vi "Programmer.vi"() -> ()   [LabVIEW 2017]
uses:
  <vilib>/Utility/config.llb/Read Key (String).vi
  <vilib>/Instr/_visa.llb/VISA Configure Serial Port (Instr).vi
  <vilib>/Utility/config.llb/NI_LVConfig.lvlib
panel:
  in  "CmdBaud":u32(ring)=230400 items=["4800"=4800, "9600"=9600, "19200"=19200, "38400"=38400, "57600"=57600, "115200"=115200, "230400"=230400, "460800"=460800, "921600"=921600]
  in  "FlashBaud":u32(ring)=230400 items=["4800"=4800, "9600"=9600, "19200"=19200, "38400"=38400, "57600"=57600, "115200"=115200, "230400"=230400, "460800"=460800, "921600"=921600]
  in  "COM Port":refnum<visa-resource-name>="COM4"
  out "RxMessage":u8[](array[numeric])
  out "LoaderCmdCount":i32
  in  "ClearPannel":bool
  in  "Read":bool
  out "Timeout?":bool
  out "Error List":string
  in  "Start":bool
  out "HeaderCount":i32
  out "AutoBaudCount":i32
  in  "File Path Control":path
  in  "Connect":bool
  in  "Stop Button":bool
  out "Rx":u64
  out "Tx":u64
  # "Ver 1.0.7"
  # "© Redler Technologies. All Rights Reserved"
  # "16:20:49 Operation stopped by user\n16:20:15 Driver Version: 20215\n16:20:14 Getting Driver version...\n16:20:14 Program success !\n16:20:13 Program start...\n16:20:13 Erase success !\n16:20:08 Erase start...\n16:20:08 Autobaud handshake success !\n16:20:05 Sending autobaud operation...\n16:20:05 Getting Driver version failed !\n16:20:02 Getting Driver version...\n16:20:02 Openning COM Port success !\n16:20:01 Openning COM Port..."
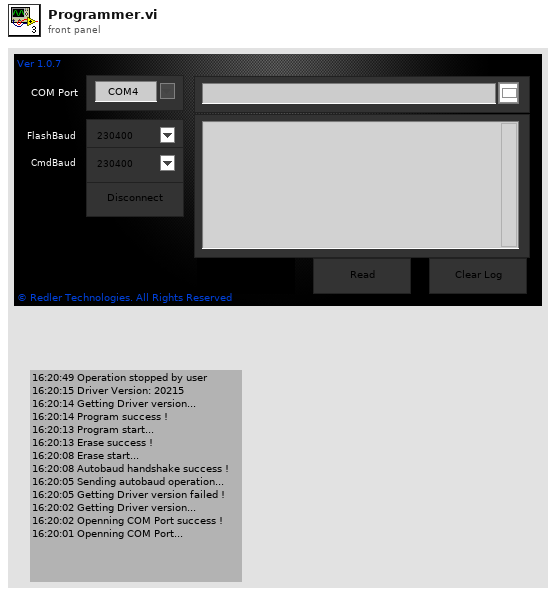
[diagram p1: front panel]
types:
  T1 = typedef "Semaphore RefNum" = refnum<k1>
  T2 = cluster{"Send Debug":string, "idx":i32, "DataType":enum8{"Int", " float"}, "Cmd id":u16, "Get/Set":enum8{"Set", "Get"}}
  T3 = cluster{"Send Debug":string, "idx":u16, "DataType":enum8{"Int", " float"}, "Cmd id":u16, "Get/Set":enum8{"Set", "Get"}}
  T4 = cluster{"Send Debug":string, "idx":u16, "DataType":enum8{"Int", " float"}, "Cmd id":u16, "Get/Set":enum8{"Set", "Get"}}[]
  T5 = typedef "NI_LVConfig.lvlib/Config Data RefNum.ctl" = refnum<k1>
  T6 = cluster{"Data":string, "idx":u16, "DataType":enum8{"Int", " float"}, "Cmd id":u16, "Get/Set":enum8{"Set", "Get"}}
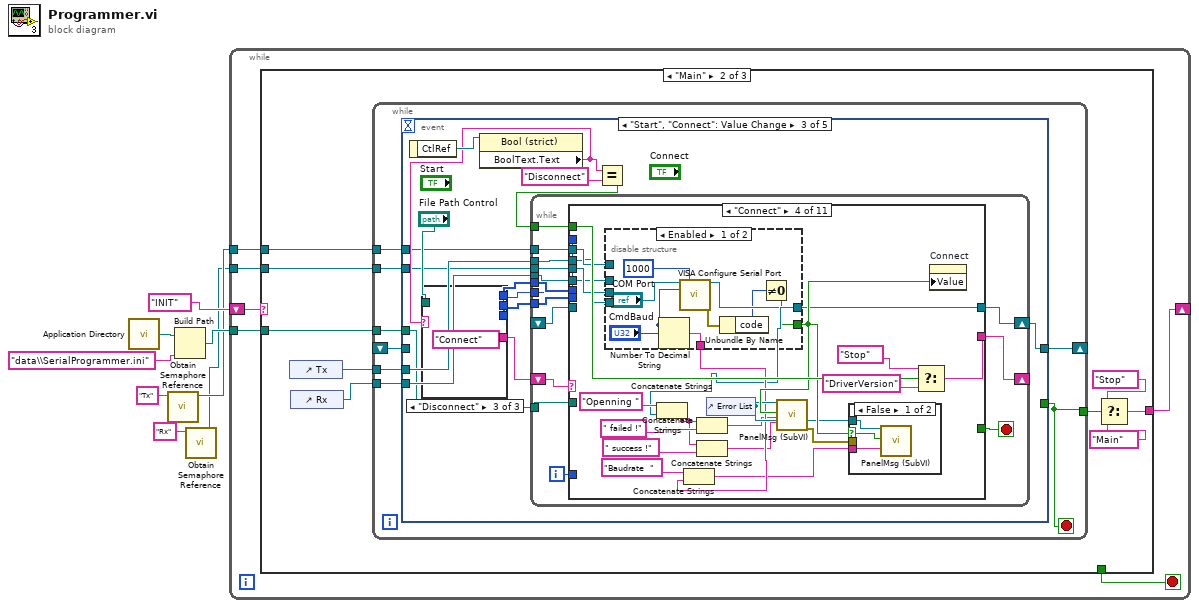
[diagram p0: block diagram]
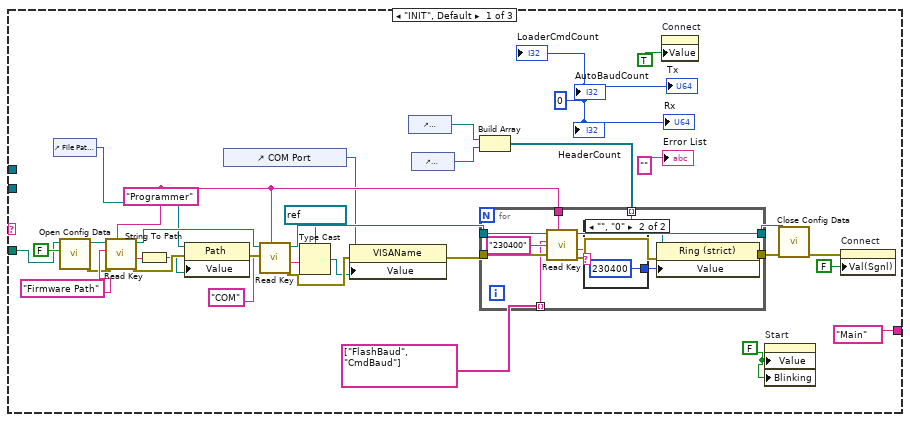
[diagram p2: hidden frame]
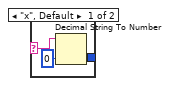
[diagram p3: hidden frame]
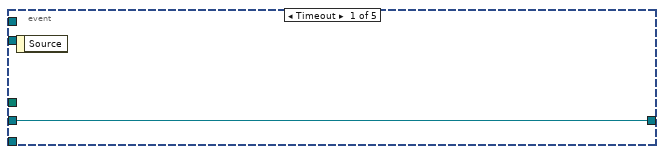
[diagram p4: hidden frame]
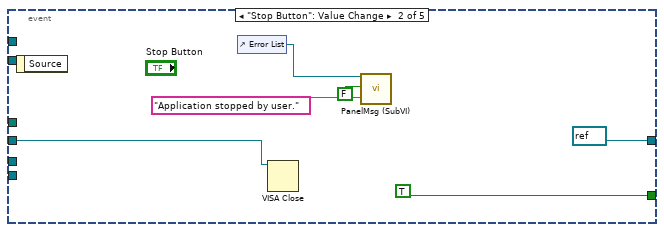
[diagram p5: hidden frame]
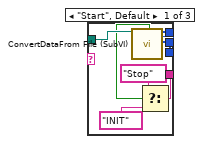
[diagram p6: hidden frame]
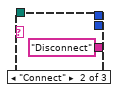
[diagram p7: hidden frame]
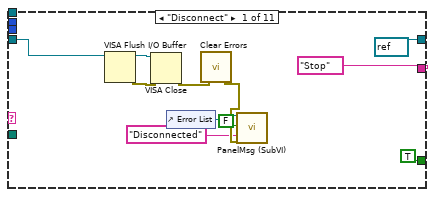
[diagram p8: hidden frame]
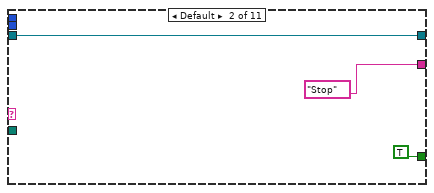
[diagram p9: hidden frame]
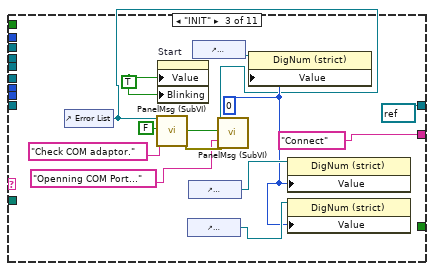
[diagram p10: hidden frame]
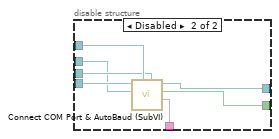
[diagram p12: hidden frame]
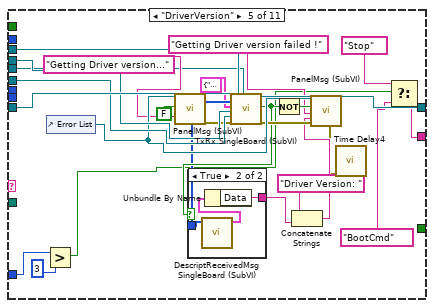
[diagram p13: hidden frame]
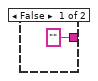
[diagram p14: hidden frame]
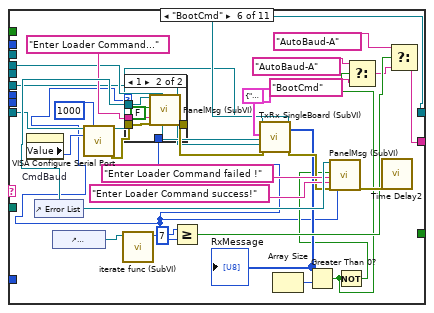
[diagram p15: hidden frame]
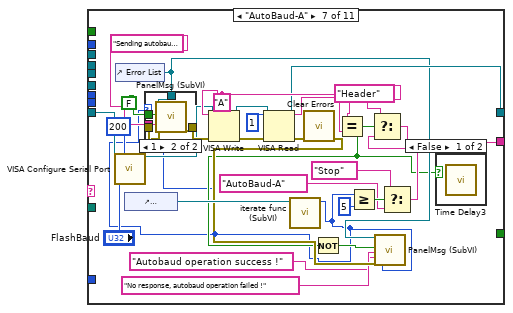
[diagram p17: hidden frame]
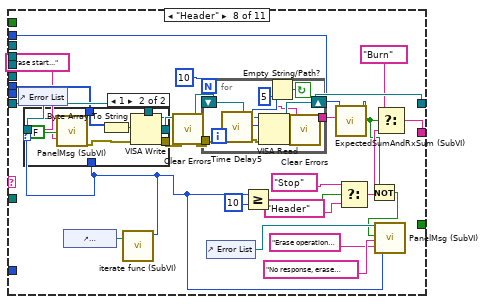
[diagram p20: hidden frame]
diagram:
  n1 = call <vilib>:"Application Directory.vi"() -> ("Application Directory"=w7:path)
  n2 = call <vilib>:"Obtain Semaphore Reference.vi"("name (unnamed)"="Tx") -> ("semaphore"=w2:T1)  [unwired: 4 in, 2 out]
  n3 = Build Path(base path=w7, name or relative path="data\\SerialProgrammer.ini") -> (appended path=w5:path)
  n4 = call <vilib>:"Obtain Semaphore Reference.vi"("name (unnamed)"="Rx") -> ("semaphore"=w1:T1)  [unwired: 4 in, 2 out]
  n5 = while {
    shift-right: [w12] -> _
    shift-left: "INIT" ("Combo Box") -> [w14]
    tunnel: w5 -> [w11]
    tunnel: w2 -> [w10]
    tunnel: w1 -> [w9]
    stop <- w13 stop-if-true
    n6 = case shown="\"Main\"" w14 {
      tunnel: [_ _ TRUE] -> w13
      tunnel: ["Main" ("Combo Box") w66 "Stop" ("Combo Box")] -> w12
      tunnel: w11 -> [w24 w65 _]
      tunnel: w10 -> [_ w64 _]
      tunnel: w9 -> [_ w63 _]
      frame "INIT", Default {
        w22 = FALSE ("Start")
        w33 = "Programmer" ("section")
        w21 = 0 ("AutoBaudCount")
        n7 = control-ref of="File Path Control"() -> (w30:refnum<vi>)
        n8 = call <vilib>:"Open Config Data.vi"("create file if necessary (T)"=FALSE, "configuration file path"=w24) -> ("error out"=w23:errorcluster, "refnum"=w25:T5)  [unwired: 1 in, 7 out]
        n9 = call-poly <vilib>:"Read Key.vi"("section"=w33, "error in (no error)"=w23, "key"="Firmware Path", "refnum"=w25) -> ("error out"=w40:errorcluster, "value"=w28:string, "refnum out"=w38:T5)  [unwired: 2 in, 3 out]
        n10 = String To Path(string=w28) -> (path=w27:path)
        n11 = property on="Property Node" class="Path"(reference=w30, error in=w40, "Value"=w27) -> (error out=w39:errorcluster)  [unwired: 1 out]
        n12 = control-ref of="COM Port"() -> (w29:refnum<vi>)
        n13 = call-poly <vilib>:"Read Key.vi"("section"=w33, "error in (no error)"=w39, "key"="COM", "refnum"=w38) -> ("error out"=w42:errorcluster, "value"=w36:string, "refnum out"=w35:T5)  [unwired: 2 in, 3 out]
        n14 = Type Cast(type=refnum<visa-resource-name> "COM1" ("UUT COM Port 2"), x=w36) -> (*(type *) &x=w37:refnum<visa-resource-name>)
        n15 = property on="Property Node" class="VISAName"(reference=w29, error in=w42, "Value"=w37) -> (error out=w43:errorcluster)  [unwired: 1 out]
        n16 = control-ref of="FlashBaud"() -> (w20:refnum<vi>)
        n17 = control-ref of="CmdBaud"() -> (w19:refnum<vi>)
        n18 = Build Array(w20, w19) -> (w18:refnum<vi>[])
        n19 = for {
          tunnel: w33 -> [w52]
          tunnel: w43 -> [w56]
          tunnel: [w58] -> w44
          tunnel: w35 -> [w53]
          tunnel: [w55] -> w41
          tunnel: w18 -> [w50] mode=indexing
          tunnel: string[] ["FlashBaud", "CmdBaud"] -> [w49] mode=indexing
          n20 = call-poly <vilib>:"Read Key.vi"("section"=w52, "error in (no error)"=w56, "default value"="230400", "key"=w49, "refnum"=w53) -> ("error out"=w57:errorcluster, "value"=w48:string, "refnum out"=w55:T5)  [unwired: 1 in, 3 out]
          n21 = case shown="\"\", \"0\"" w48 {
            selector: w48 -> [w59 _]
            tunnel: [w61 u32 230400] -> w54
            frame "x", Default {
              n22 = Decimal String To Number(string=w59, default (0L)=u32 0 ("default (0 I32)")) -> (number=w61:u32)  [unwired: 1 in, 1 out]
            }
            frame "", "0" {
            }
          }
          n23 = property on="Property Node" class="Ring (strict)"(reference=w50, error in=w57, "Value"=w54) -> (error out=w58:errorcluster)  [unwired: 1 out]
        }
        n24 = property on="Connect" class="Bool (strict)"("Value"=TRUE ("Connect")) -> ()  [unwired: 2 in, 2 out]
        n25 = property on="Start" class="Bool (strict)"("Value"=w22, "Blinking"=w22) -> ()  [unwired: 2 in, 2 out]
        n26 = call <vilib>:"Close Config Data.vi"("error in (no error)"=w44, "refnum"=w41) -> ("error out"=w15:errorcluster)  [unwired: 1 in, 8 out]
        n27 = property on="Connect" class="Bool (strict)"(error in=w15, "Val(Sgnl)"=FALSE ("Value (Signaling)")) -> ()  [unwired: 1 in, 2 out]
        "Tx" <- w21
        "Rx" <- w21
        "AutoBaudCount" <- w21
        "HeaderCount" <- w21
        "Error List" <- "" ("Error List")
        "LoaderCmdCount" <- w21
      }
      frame "Main" {
        n28 = control-ref of="Tx"() -> (w71:refnum<vi>)
        n29 = control-ref of="Rx"() -> (w70:refnum<vi>)
        n30 = while {
          shift-right: [w79] -> _
          shift-left: _ -> [w78]
          tunnel: w70 -> [w77]
          tunnel: w71 -> [w76]
          tunnel: [w75] -> w69
          tunnel: w65 -> [w74]
          tunnel: w64 -> [w73]
          tunnel: w63 -> [w72]
          stop <- w75 stop-if-true
          n31 = event shown="[2] \"Start\", \"Connect\": Value Change" {
            selector: _ -> [_ _ _ _ _]
            dyn-events: _ -> [_ _ _ _ _]
            timeout: _ -> [_ _ _ _ _]
            tunnel: [_ TRUE _ _ _] -> w75
            tunnel: [w80 refnum<visa-resource-name> refnum ("VISA Refnum out") w96 w371 w381] -> w79
            tunnel: w78 -> [w80 w85 _ w371 w383]
            tunnel: w77 -> [_ _ w97 _ w384]
            tunnel: w76 -> [_ _ w98 _ w385]
            tunnel: w74 -> [_ _ w89 _ _]
            tunnel: w73 -> [_ _ w88 _ w379]
            tunnel: w72 -> [_ _ w87 _ w378]
            event Timeout {
              n32 = event-data() -> ()  [unwired: 1 in, 1 out]
            }
            event "Stop Button": Value Change {
              n33 = event-data() -> ()  [unwired: 1 in, 1 out]
              n34 = control-ref of="Error List"() -> (w83:refnum<vi>)
              n35 = VISA Close(VISA resource name=w85) -> ()  [unwired: 1 in, 1 out]
              n36 = call "PanelMsg (SubVI).vi"("Pannel Messages"=w83, "Error?(T)"=FALSE, "OKMsg"="Application stopped by user.") -> ()  [unwired: 16 in, 1 out]
            }
            event "Start", "Connect": Value Change {
              n37 = event-data() -> ("CtlRef"=w94:refnum<vi>)  [unwired: 1 in]
              n38 = property class="Bool (strict)"(reference=w94) -> ("BoolText.Text"=w90:string)  [unwired: 1 in, 2 out]
              n39 = case shown="\"Disconnect\"" w90 {
                tunnel: [w109 _ _] -> w101
                tunnel: [w108 _ _] -> w100
                tunnel: [w107 _ _] -> w99
                tunnel: "File Path Control" -> [w106 _ _]
                tunnel: [w102 "Disconnect" ("Combo Box") "Connect" ("Combo Box")] -> w95
                frame "Start", Default {
                  n40 = call "ConvertDataFrom File (SubVI).vi"("File Path Control"=w106) -> ("WrongFile?"=w105:bool, "Header"=w107:u8[], "sumHeader"=w108:u16, "Full Text File"=w109:u8[])  [unwired: 13 in, 2 out]
                  n41 = Select(t="Stop" ("Combo Box"), s=w105, f="INIT" ("Combo Box")) -> (s? t:f=w102:string)
                }
                frame "Connect" {
                }
                frame "Disconnect" {
                }
              }
              n42 = Equal?(x=w90, y="Disconnect") -> (x = y?=w92:bool)
              n43 = while {
                shift-right: [w126] -> _
                shift-left: w95 -> [w117]
                shift-right: [w125] -> w96
                shift-left: _ -> [w124]
                tunnel: w98 -> [w123]
                tunnel: w97 -> [w122]
                tunnel: w99 -> [w120]
                tunnel: w100 -> [w119]
                tunnel: w101 -> [w118]
                tunnel: w92 -> [w116]
                tunnel: w89 -> [w115]
                tunnel: w88 -> [w113]
                tunnel: w87 -> [w112]
                i -> [w114]
                stop <- w121 stop-if-true
                n44 = case shown="\"Connect\"" w117 {
                  tunnel: ["Stop" ("Combo Box") "Stop" ("Combo Box") "Connect" ("Combo Box") w171 w199 w249 w270 w307 w337 "DriverVersion" ("Combo Box") "Stop" ("Combo Box")] -> w126
                  tunnel: [refnum<visa-resource-name> refnum ("VISA resource name out") w140 refnum<visa-resource-name> refnum ("VISA Refnum out") w153 w214 w231 w281 w315 w347 w354 w366] -> w125
                  tunnel: w124 -> [w132 w140 _ _ w217 w226 w259 w316 w347 w356 w366]
                  tunnel: w123 -> [_ _ _ w166 w216 w235 _ _ _ _ _]
                  tunnel: w122 -> [_ _ _ w165 w215 w234 _ _ _ _ _]
                  tunnel: [TRUE TRUE _ _ _ _ _ _ _ _ TRUE] -> w121
                  tunnel: w120 -> [_ _ _ _ _ _ _ w313 _ _ _]
                  tunnel: w119 -> [_ _ _ _ _ _ _ w306 _ _ _]
                  tunnel: w118 -> [_ _ _ _ _ _ _ _ w352 _ _]
                  tunnel: w116 -> [_ _ _ w172 _ _ _ _ _ _ _]
                  tunnel: w115 -> [_ _ _ _ _ _ _ _ _ _ w361]
                  tunnel: w114 -> [_ _ _ _ w195 _ _ _ _ _ _]
                  tunnel: w113 -> [_ _ _ w168 w193 _ _ _ _ _ _]
                  tunnel: w112 -> [_ _ _ w167 w192 _ _ _ _ _ _]
                  frame "Disconnect" {
                    n45 = VISA Flush I/O Buffer(VISA resource name=w132) -> (VISA resource name out=w135:refnum<visa-resource-name>, error out=w134:errorcluster)  [unwired: 2 in]
                    n46 = VISA Close(VISA resource name=w135, error in (no error)=w134) -> (error out=w133:errorcluster)
                    n47 = control-ref of="Error List"() -> (w131:refnum<vi>)
                    n48 = call <vilib>:"Clear Errors.vi"("error in (no error)"=w133) -> ("error out"=w130:errorcluster)  [unwired: 5 in, 1 out]
                    n49 = call "PanelMsg (SubVI).vi"("Pannel Messages"=w131, "Error?(T)"=FALSE, "OKMsg"="Disconnected", "error in (no error)"=w130) -> ()  [unwired: 15 in, 1 out]
                  }
                  frame Default {
                  }
                  frame "INIT" {
                    w143 = FALSE ("Error?(T)")
                    w145 = 0 ("Value")
                    w150 = TRUE ("Start")
                    n50 = control-ref of="Error List"() -> (w144:refnum<vi>)
                    n51 = call "PanelMsg (SubVI).vi"("Pannel Messages"=w144, "Error?(T)"=w143, "OKMsg"="Check COM adaptor.") -> ("error out"=w142:errorcluster)  [unwired: 16 in]
                    n52 = property on="Start" class="Bool (strict)"("Value"=w150, "Blinking"=w150) -> ()  [unwired: 2 in, 2 out]
                    n53 = control-ref of="HeaderCount"() -> (w146:refnum<vi>)
                    n54 = control-ref of="LoaderCmdCount"() -> (w147:refnum<vi>)
                    n55 = control-ref of="AutoBaudCount"() -> (w149:refnum<vi>)
                    n56 = call "PanelMsg (SubVI).vi"("Pannel Messages"=w144, "Error?(T)"=w143, "OKMsg"="Openning COM Port...", "error in (no error)"=w142) -> ()  [unwired: 15 in, 1 out]
                    n57 = property class="DigNum (strict)"(reference=w149, "Value"=w145) -> ()  [unwired: 1 in, 2 out]
                    n58 = property class="DigNum (strict)"(reference=w147, "Value"=w145) -> ()  [unwired: 1 in, 2 out]
                    n59 = property class="DigNum (strict)"(reference=w146, "Value"=w145) -> ()  [unwired: 1 in, 2 out]
                  }
                  frame "Connect" {
                    n60 = disable-structure shown="Enabled" {
                      disable-tunnel: [w184 w185] -> w153
                      disable-tunnel: [w177 w187] -> w170
                      disable-tunnel: w168 -> [_ w191]
                      disable-tunnel: w167 -> [_ w190]
                      disable-tunnel: w166 -> [_ w189]
                      disable-tunnel: w165 -> [_ w188]
                      disable-tunnel: [w179 w186] -> w162
                      frame Enabled {
                        n61 = Number To Decimal String(number="CmdBaud") -> (decimal integer string=w179:string)  [unwired: 1 in]
                        n62 = call-poly "VISA Configure Serial Port"("VISA resource name"="COM Port", "timeout (10sec)"=u32 1000, "baud rate (9600)"="CmdBaud") -> ("VISA resource name out"=w184:refnum<visa-resource-name>, "error out"=w181:errorcluster)  [unwired: 11 in]
                        n63 = Unbundle By Name(w181) -> ("code"=w178:i32)
                        n64 = Not Equal To 0?(x=w178) -> (x != 0?=w177:bool)
                      }
                      frame Disabled {
                        n65 = call "Connect COM Port & AutoBaud (SubVI).vi"("Rx semaphore"=w190, "Tx semaphore"=w191, "Rx"=w188, "Tx"=w189) -> ("BaudRate"=w186:string, "Success?"=w187:bool, "VISA Refnum out"=w185:refnum<visa-resource-name>)  [unwired: 4 in, 1 out]
                      }
                    }
                    n66 = Concatenate Strings("Openning ", w153) -> (w158:string)
                    n67 = Concatenate Strings("Baudrate  ", w162) -> (w161:string)
                    n68 = Concatenate Strings(w158, " failed !" ("string")) -> (w155:string)
                    n69 = Concatenate Strings(w158, " success !" ("string")) -> (w156:string)
                    n70 = control-ref of="Error List"() -> (w164:refnum<vi>)
                    n71 = call "PanelMsg (SubVI).vi"("Pannel Messages"=w164, "Error?(T)"=w170, "ErrorMsg"=w155, "OKMsg"=w156) -> ("error out"=w154:errorcluster)  [unwired: 15 in]
                    n72 = case shown="False" w170 {
                      selector: w170 -> [w175 _]
                      tunnel: w164 -> [w176 _]
                      tunnel: w161 -> [w174 _]
                      tunnel: w154 -> [_ _]
                      frame False {
                        n73 = call "PanelMsg (SubVI).vi"("Pannel Messages"=w176, "Error?(T)"=w175, "OKMsg"=w174) -> ()  [unwired: 16 in, 1 out]
                      }
                      frame True {
                      }
                    }
                    n74 = Select(t="Stop" ("Combo Box"), s=w172, f="DriverVersion") -> (s? t:f=w171:string)
                    n75 = property on="Connect" class="Bool (strict)"("Value"=w170) -> ()  [unwired: 2 in, 2 out]
                  }
                  frame "DriverVersion" {
                    n76 = Greater?(x=w195, y=3 ("x")) -> (0:w196:bool)
                    n77 = control-ref of="Error List"() -> (w213:refnum<vi>)
                    n78 = call "PanelMsg (SubVI).vi"("Pannel Messages"=w213, "Error?(T)"=FALSE, "OKMsg"="Getting Driver version...") -> ("error out"=w211:errorcluster)  [unwired: 16 in]
                    n79 = call "TxRx SingleBoard (SubVI).vi"("VISA Refnum in"=w217, "DataMessage Tx"=T2 {"Send Debug"="", "idx"=4, "DataType"=enum."Int", "Cmd id"=62, "Get/Set"=enum."Get"}, "Tx"=w216, "Rx"=w215, "error in (no error)"=w211, "Tx semaphore"=w193, "Rx semaphore"=w192) -> ("VISA Refnum out"=w214:refnum<visa-resource-name>, "RxMessage"=w205:u8[], "DataReceived?"=w208:bool, "error out"=w212:errorcluster)  [unwired: 6 in, 3 out]
                    n80 = case shown="True" w208 {
                      tunnel: ["" ("Data") w220] -> w207
                      tunnel: w205 -> [_ w219]
                      frame False {
                      }
                      frame True {
                        n81 = call "DescriptReceivedMsg SingleBoard (SubVI).vi"("RxMessageArray"=w219) -> ("DataMessage Rx"=w221:T6)  [unwired: 9 in, 1 out]
                        n82 = Unbundle By Name(w221) -> ("Data"=w220:string)
                      }
                    }
                    n83 = Not(x=w208) -> (.not. x?=w209:bool)
                    n84 = Concatenate Strings("Driver Version: ", w207) -> (w206:string)
                    n85 = call "PanelMsg (SubVI).vi"("Pannel Messages"=w213, "Error?(T)"=w209, "ErrorMsg"="Getting Driver version failed !", "OKMsg"=w206, "error in (no error)"=w212) -> ("error out"=w204:errorcluster)  [unwired: 14 in]
                    n86 = call "Time Delay4"("error in (no error)"=w204) -> ()  [unwired: 10 in, 1 out]
                    n87 = Select(t="Stop" ("Combo Box"), s=w196, f="BootCmd" ("Combo Box")) -> (s? t:f=w199:string)
                  }
                  frame "BootCmd" {
                    n88 = property on="CmdBaud" class="Ring (strict)"() -> ("Value"=w223:u32)  [unwired: 2 in, 2 out]
                    n89 = control-ref of="Error List"() -> (w250:refnum<vi>)
                    n90 = control-ref of="LoaderCmdCount"() -> (w242:refnum<vi>)
                    n91 = call-poly "VISA Configure Serial Port"("VISA resource name"=w226, "timeout (10sec)"=u32 1000, "baud rate (9600)"=w223) -> ("VISA resource name out"=w225:refnum<visa-resource-name>, "error out"=w224:errorcluster)  [unwired: 11 in]
                    n92 = call "iterate func (SubVI).vi"("int i; Ref"=w242) -> ("Actual Value (i)"=w222:i32)  [unwired: 10 in]
                    n93 = case shown="1" w222 {
                      tunnel: w250 -> [_ w256]
                      tunnel: [w251 w255] -> w248
                      tunnel: "Enter Loader Command..." -> [_ w253]
                      tunnel: w224 -> [w251 w252]
                      tunnel: w222 -> [_ _]
                      frame 2, Default {
                      }
                      frame 1 {
                        n94 = call "PanelMsg (SubVI).vi"("Pannel Messages"=w256, "Error?(T)"=FALSE, "OKMsg"=w253, "error in (no error)"=w252) -> ("error out"=w255:errorcluster)  [unwired: 15 in]
                      }
                    }
                    n95 = Greater Or Equal?(x=w222, y=7) -> (x >= y?=w240:bool)
                    n96 = call "TxRx SingleBoard (SubVI).vi"("VISA Refnum in"=w225, "DataMessage Tx"=T3 {"Send Debug"="1", "idx"=0, "DataType"=enum."Int", "Cmd id"=65, "Get/Set"=enum."Set"}, "Tx"=w235, "Rx"=w234, "error in (no error)"=w248) -> ("VISA Refnum out"=w231:refnum<visa-resource-name>, "RxMessage"=w230:u8[], "error out"=w232:errorcluster)  [unwired: 8 in, 4 out]
                    "RxMessage" <- w230
                    n97 = Array Size(array=w230) -> (size(s)=w233:i32)
                    n98 = Greater Than 0?(x=w233) -> (x > 0?=w228:bool)
                    n99 = Not(x=w228) -> (.not. x?=w229:bool)
                    n100 = call "PanelMsg (SubVI).vi"("Pannel Messages"=w250, "Error?(T)"=w229, "ErrorMsg"="Enter Loader Command failed !", "OKMsg"="Enter Loader Command success!", "error in (no error)"=w232, "Iterrator"=w222) -> ("error out"=w247:errorcluster)  [unwired: 13 in]
                    n101 = Select(t="AutoBaud-A" ("Combo Box"), s=w228, f="BootCmd" ("Combo Box")) -> (s? t:f=w237:string)
                    n102 = call "Time Delay2"("error in (no error)"=w247) -> ()  [unwired: 10 in, 1 out]
                    n103 = Select(t="AutoBaud-A" ("Combo Box"), s=w240, f=w237) -> (s? t:f=w249:string)
                  }
                  frame "AutoBaud-A" {
                    w283 = "A" ("write buffer")
                    n104 = call-poly "VISA Configure Serial Port"("VISA resource name"=w259, "timeout (10sec)"=u32 200, "baud rate (9600)"="FlashBaud") -> ("VISA resource name out"=w261:refnum<visa-resource-name>, "error out"=w258:errorcluster)  [unwired: 11 in]
                    n105 = control-ref of="Error List"() -> (w268:refnum<vi>)
                    n106 = control-ref of="AutoBaudCount"() -> (w279:refnum<vi>)
                    n107 = call "iterate func (SubVI).vi"("int i; Ref"=w279) -> ("Actual Value (i)"=w257:i32)  [unwired: 10 in]
                    n108 = case shown="1" w257 {
                      tunnel: [w287 w292] -> w273
                      tunnel: FALSE ("Error?(T)") -> [_ w291]
                      tunnel: "Sending autobaud operation..." -> [_ w290]
                      tunnel: w268 -> [_ w289]
                      tunnel: w258 -> [w287 w288]
                      tunnel: w257 -> [_ _]
                      frame 2, Default {
                      }
                      frame 1 {
                        n109 = call "PanelMsg (SubVI).vi"("Pannel Messages"=w289, "Error?(T)"=w291, "OKMsg"=w290, "error in (no error)"=w288) -> ("error out"=w292:errorcluster)  [unwired: 15 in]
                      }
                    }
                    n110 = VISA Write(VISA resource name=w261, write buffer=w283, error in (no error)=w273) -> (VISA resource name out=w285:refnum<visa-resource-name>, error out=w263:errorcluster)  [unwired: 1 out]
                    n111 = VISA Read(VISA resource name=w285, byte count=u32 1, error in (no error)=w263) -> (VISA resource name out=w281:refnum<visa-resource-name>, read buffer=w284:string, error out=w280:errorcluster)  [unwired: 1 out]
                    n112 = call <vilib>:"Clear Errors.vi"("error in (no error)"=w280) -> ("error out"=w269:errorcluster)  [unwired: 5 in, 1 out]
                    n113 = Equal?(x=w284, y=w283) -> (x = y?=w267:bool)
                    n114 = Not(x=w267) -> (.not. x?=w266:bool)
                    n115 = Greater Or Equal?(x=w257, y=5) -> (x >= y?=w277:bool)
                    n116 = call "PanelMsg (SubVI).vi"("Pannel Messages"=w268, "Error?(T)"=w266, "ErrorMsg"="No response, autobaud operation failed !" ("string"), "OKMsg"="Autobaud operation success !", "error in (no error)"=w269, "Iterrator"=w257) -> ()  [unwired: 13 in, 1 out]
                    n117 = Select(t="Stop" ("Combo Box"), s=w277, f="AutoBaud-A" ("Combo Box")) -> (s? t:f=w275:string)
                    n118 = Select(t="Header" ("Combo Box"), s=w267, f=w275) -> (s? t:f=w270:string)
                    n119 = case shown="False" w267 {
                      frame False {
                        n120 = call "Time Delay3"() -> ()  [unwired: 11 in, 1 out]
                      }
                      frame True {
                      }
                    }
                  }
                  frame "Header" {
                    n121 = control-ref of="Error List"() -> (w301:refnum<vi>)
                    n122 = control-ref of="HeaderCount"() -> (w303:refnum<vi>)
                    n123 = call "iterate func (SubVI).vi"("int i; Ref"=w303) -> ("Actual Value (i)"=w293:i32)  [unwired: 10 in]
                    n124 = case shown="1" w293 {
                      tunnel: [w318 w328] -> w317
                      tunnel: w316 -> [w318 w327]
                      tunnel: [errorcluster {"status"=FALSE, "code"=0, "source"=""} ("error out") w326] -> w314
                      tunnel: w313 -> [_ w325]
                      tunnel: "Erase start..." -> [_ w323]
                      tunnel: w301 -> [_ w322]
                      tunnel: w293 -> [_ _]
                      frame 2, Default {
                      }
                      frame 1 {
                        n125 = call "PanelMsg (SubVI).vi"("Pannel Messages"=w322, "Error?(T)"=FALSE, "OKMsg"=w323) -> ("error out"=w321:errorcluster)  [unwired: 16 in]
                        n126 = Byte Array To String(unsigned byte array=w325) -> (string=w320:string)
                        n127 = VISA Write(VISA resource name=w327, write buffer=w320, error in (no error)=w321) -> (VISA resource name out=w328:refnum<visa-resource-name>, error out=w326:errorcluster)  [unwired: 1 out]
                      }
                    }
                    n128 = call <vilib>:"Clear Errors.vi"("error in (no error)"=w314) -> ("error out"=w295:errorcluster)  [unwired: 5 in, 1 out]
                    n129 = for {
                      N: 10 -> [_]
                      tunnel: [w330] -> w305
                      tunnel: w295 -> [w332]
                      shift-right: [w333] -> w315
                      shift-left: w317 -> [w335]
                      stop <- w329 continue-if-true
                      n130 = call "Time Delay5"("error in (no error)"=w332) -> ("error out"=w331:errorcluster)  [unwired: 10 in]
                      n131 = VISA Read(VISA resource name=w335, byte count=u32 5, error in (no error)=w331) -> (VISA resource name out=w333:refnum<visa-resource-name>, read buffer=w330:string, error out=w334:errorcluster)  [unwired: 1 out]
                      n132 = Empty String/Path?(string/path=w330) -> (empty?=w329:bool)
                      n133 = call <vilib>:"Clear Errors.vi"("error in (no error)"=w334) -> ()  [unwired: 5 in, 2 out]
                    }
                    n134 = control-ref of="Error List"() -> (w300:refnum<vi>)
                    n135 = Greater Or Equal?(x=w293, y=10) -> (x >= y?=w311:bool)
                    n136 = call "ExpectedSumAndRxSum (SubVI).vi"("Header in"=w305, "Numeric Control"=w306) -> ("Equal?"=w297:bool)  [unwired: 9 in]
                    n137 = Select(t="Stop" ("Combo Box"), s=w311, f="Header" ("Combo Box")) -> (s? t:f=w308:string)
                    n138 = Not(x=w297) -> (.not. x?=w296:bool)
                    n139 = call "PanelMsg (SubVI).vi"("Pannel Messages"=w300, "Error?(T)"=w296, "ErrorMsg"="No response, erase operation failed !" ("string"), "OKMsg"="Erase operation success !", "Iterrator"=w293) -> ()  [unwired: 14 in, 1 out]
                    n140 = Select(t="Burn" ("Combo Box"), s=w297, f=w308) -> (s? t:f=w307:string)
                  }
                  frame "Burn" {
                    n141 = control-ref of="Error List"() -> (w346:refnum<vi>)
                    n142 = call "PanelMsg (SubVI).vi"("Pannel Messages"=w346, "Error?(T)"=FALSE, "OKMsg"="Program start...") -> ("error out"=w351:errorcluster)  [unwired: 16 in]
                    n143 = call "LoadData (SubVI).vi"("error in (no error)"=w351, "VISA resource name out"=w347, "Full Text File"=w352) -> ("error out"=w348:errorcluster, "Timeout?"=w340:bool)  [unwired: 4 in, 3 out]
                    "Timeout?" <- w340
                    n144 = call <vilib>:"Clear Errors.vi"("error in (no error)"=w348) -> ("error out"=w341:errorcluster)  [unwired: 5 in, 1 out]
                    n145 = call "PanelMsg (SubVI).vi"("Pannel Messages"=w346, "Error?(T)"=w340, "ErrorMsg"="Program failed !" ("string"), "OKMsg"="Program success !" ("string"), "error in (no error)"=w341) -> ("error out"=w343:errorcluster)  [unwired: 14 in]
                    n146 = call <vilib>:"Clear Errors.vi"("error in (no error)"=w343) -> ("error out"=w342:errorcluster)  [unwired: 5 in, 1 out]
                    n147 = call "Time Delay6"("error in (no error)"=w342) -> ()  [unwired: 10 in, 1 out]
                    n148 = Select(t="Stop", s=w340, f="Reconnect" ("Combo Box")) -> (s? t:f=w337:string)
                  }
                  frame "Reconnect" {
                    n149 = VISA Close(VISA resource name=w356) -> (error out=w358:errorcluster)  [unwired: 1 in]
                    n150 = call <vilib>:"Clear Errors.vi"("error in (no error)"=w358) -> ("error out"=w355:errorcluster)  [unwired: 5 in, 1 out]
                    n151 = property on="CmdBaud" class="Ring (strict)"() -> ("Value"=w353:u32)  [unwired: 2 in, 2 out]
                    n152 = call-poly "VISA Configure Serial Port"("VISA resource name"=w356, "timeout (10sec)"=u32 1000, "baud rate (9600)"=w353, "error in (no error)"=w355) -> ("VISA resource name out"=w354:refnum<visa-resource-name>)  [unwired: 10 in, 1 out]
                  }
                  frame "Stop" {
                    w365 = FALSE ("Start")
                    n153 = control-ref of="File Path Control"() -> (w362:refnum<vi>)
                    n154 = control-ref of="FlashBaud"() -> (w360:refnum<vi>)
                    n155 = control-ref of="CmdBaud"() -> (w364:refnum<vi>)
                    n156 = control-ref of="COM Port"() -> (w363:refnum<vi>)
                    n157 = call "Save SerialParameters (SubVI).vi"("FlashBaud"=w360, "appended path"=w361, "CmdBaud"=w364, "COM Port"=w363, "Path in"=w362) -> ()  [unwired: 7 in]
                    n158 = property on="Start" class="Bool (strict)"("Value"=w365, "Blinking"=w365) -> ()  [unwired: 2 in, 2 out]
                  }
                }
              }
            }
            event "ClearPannel": Value Change {
              n159 = event-data() -> ()  [unwired: 1 in, 6 out]
              n160 = property on="ClearPannel" class="Bool (strict)"("Value"=FALSE ("ClearPannel")) -> ()  [unwired: 2 in, 2 out]
              n161 = control-ref of="Error List"() -> (w370:refnum<vi>)
              n162 = property class="Str"(reference=w370, "Value"="") -> ()  [unwired: 1 in, 2 out]
            }
            event "Read": Value Change {
              # "HW Ver\nSW Loader Ver\nSW Ver\nSN"
              n163 = event-data() -> ()  [unwired: 1 in, 1 out]
              n164 = property on="Read" class="Bool (strict)"("Value"=FALSE ("Read")) -> ()  [unwired: 2 in, 2 out]
              n165 = for {
                tunnel: w385 -> [w406]
                tunnel: w384 -> [w405]
                tunnel: w383 -> [w404]
                tunnel: T4 [{"Send Debug"="0", "idx"=2, "DataType"=enum."Int", "Cmd id"=62, "Get/Set"=enum."Get"}, {"Send Debug"="0", "idx"=4, "DataType"=enum."Int", "Cmd id"=62, "Get/Set"=enum."Get"}, {"Send Debug"="0", "idx"=3, "DataType"=enum."Int", "Cmd id"=62, "Get/Set"=enum."Get"}, {"Send Debug"="0", "idx"=1, "DataType"=enum."Int", "Cmd id"=62, "Get/Set"=enum."Get"}] -> [w403] mode=indexing
                tunnel: [w402] -> w381
                tunnel: string[] ["HW Version: ", "SW Loader Version: ", "SW Version: ", "SN: "] -> [w399] mode=indexing
                tunnel: w379 -> [w398]
                tunnel: w378 -> [w397]
                tunnel: [w395] -> w373 mode=indexing
                tunnel: [w394] -> w377 mode=indexing
                n166 = call "TxRx SingleBoard (SubVI).vi"("VISA Refnum in"=w404, "DataMessage Tx"=w403, "Tx"=w406, "Rx"=w405, "Tx semaphore"=w398, "Rx semaphore"=w397) -> ("VISA Refnum out"=w402:refnum<visa-resource-name>, "RxMessage"=w400:u8[])  [unwired: 7 in, 5 out]
                n167 = call "DescriptReceivedMsg SingleBoard (SubVI).vi"("RxMessageArray"=w400) -> ("error constant"=w396:errorcluster, "DataMessage Rx"=w401:T6)  [unwired: 9 in]
                n168 = Unbundle By Name(w401) -> ("Data"=w394:string)
                n169 = Concatenate Strings(w399, w394) -> (w395:string)
                n170 = call "Time Delay"("error in (no error)"=w396) -> ()  [unwired: 10 in, 1 out]
              }
              n171 = Array Max & Min(array=w377) -> (max value=w376:string, min value=w375:string)  [unwired: 2 out]
              n172 = Equal?(x=w376, y=w375) -> (x = y?=w374:bool)
              n173 = case shown="True" w374 {
                selector: w374 -> [_ w392]
                tunnel: w373 -> [w387 _]
                frame False {
                  n174 = for {
                    tunnel: w387 -> [w388] mode=indexing
                    n175 = control-ref of="Error List"() -> (w390:refnum<vi>)
                    n176 = call "PanelMsg (SubVI).vi"("Pannel Messages"=w390, "Error?(T)"=FALSE, "OKMsg"=w388) -> ()  [unwired: 16 in, 1 out]
                  }
                }
                frame True {
                  n177 = control-ref of="Error List"() -> (w393:refnum<vi>)
                  n178 = call "PanelMsg (SubVI).vi"("Pannel Messages"=w393, "Error?(T)"=w392, "ErrorMsg"="Failed reading parameters.") -> ()  [unwired: 16 in, 1 out]
                }
              }
            }
          }
        }
        n179 = Select(t="Stop" ("Combo Box"), s=w69, f="Main" ("Combo Box")) -> (s? t:f=w66:string)
      }
      frame "Stop" {
        n180 = disable-structure shown="RUN_TIME_ENGINE==True" {
          frame condition #0 (active) {
          }
          frame condition #1 {
            n181 = Quit LabVIEW(quit? (T)=TRUE) -> ()
          }
        }
      }
    }
  }
